vi "Clear.vi"(8 "error in (no error)":errorcluster, 11 "AudioGeneration in":refnum<class "AudioGeneration.lvclass">) -> (0 "error out":errorcluster)   [LabVIEW 2021, in "AudioGeneration.lvclass"]
uses:
  AudioGeneration.lvclass
  <vilib>/NI/STM/TCP/Get Connection Reference (TCP).vi
  AudioGeneration.lvclass/AudioGeneration.ctl
  <vilib>/NI/STM/NI STM.lvlib
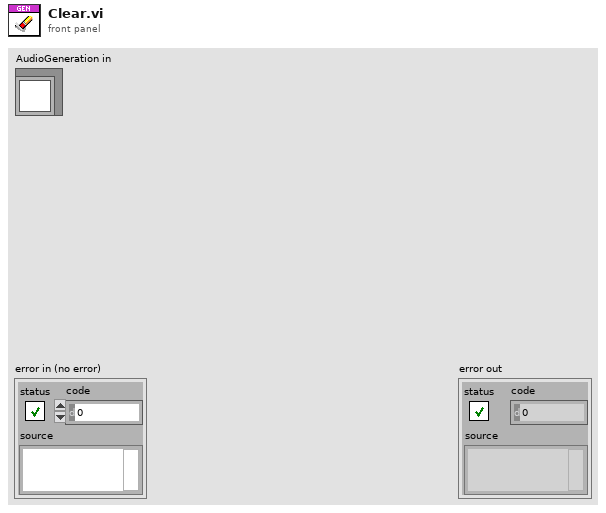
[diagram p1: front panel]
types:
  T1 = typedef "NI STM.lvlib/TCP Connection Info.ctl" = cluster{"connection ID":refnum<k5>, "meta data":T2[]}
  T2 = typedef "NI STM.lvlib/MetaDataElement.ctl" = string
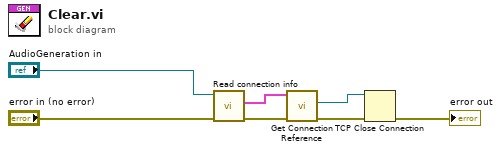
[diagram p0: block diagram]
diagram:
  n1 = call-dynamic "Read connection info.vi"("error in (no error)"="error in (no error)", "AudioGeneration in"="AudioGeneration in") -> ("error out"=w5:errorcluster, "connection info"=w4:T1)  [unwired: 7 in, 1 out]
  n2 = call-poly <vilib>:"Get Connection Reference.vi"("error in"=w5, "connection info in"=w4) -> ("error out"=w2:errorcluster, "connection ID out"=w3:refnum<k5>)  [unwired: 7 in, 1 out]
  n3 = TCP Close Connection(connection ID=w3, error in (no error)=w2) -> (error out=→"error out":errorcluster)  [unwired: 1 in, 1 out]
